vi "sub_ofdm_mes_ce.vi"(11 "ZF channel estimates":cdb[](array[numeric])) -> (3 "interpolated mes carrier CE":cdb[](array[numeric]))   [LabVIEW 2014]
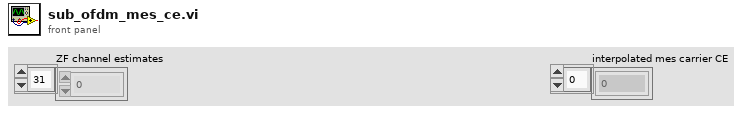
[diagram p1: front panel]
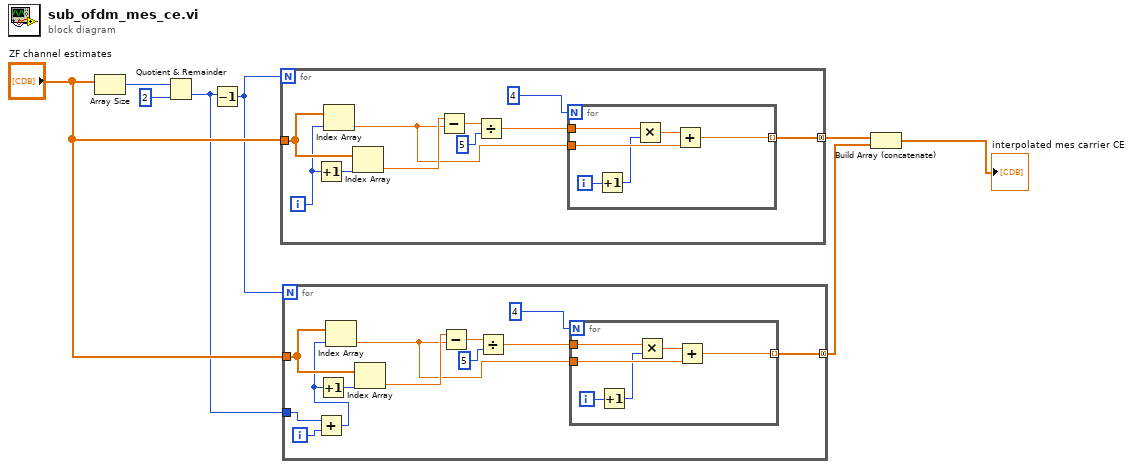
[diagram p0: block diagram]
diagram:
  n1 = Array Size(array="ZF channel estimates") -> (size(s)=w8:i32)
  n2 = Quotient & Remainder(x=w8, y=2) -> (floor(x/y)=w4:i32)  [unwired: 1 out]
  n3 = Decrement(x=w4) -> (x-1=w5:i32)
  n4 = for {
    N: w5 -> [_]
    tunnel: "ZF channel estimates" -> [w18]
    tunnel: [w9] -> w3 mode=concatenating
    i -> [w17]
    n5 = Increment(x=w17) -> (x+1=w16:i32)
    n6 = Index Array(array=w18, index=w17) -> (element=w10:cdb)
    n7 = Index Array(array=w18, index=w16) -> (element=w15:cdb)
    n8 = Subtract(x=w15, y=w10) -> (x-y=w14:cdb)
    n9 = Divide(x=w14, y=5) -> (x/y=w11:cdb)
    n10 = for {
      N: 4 -> [_]
      tunnel: w11 -> [w24]
      tunnel: w10 -> [w22]
      tunnel: [w19] -> w9 mode=indexing
      i -> [w21]
      n11 = Increment(x=w21) -> (x+1=w20:i32)
      n12 = Multiply(x=w24, y=w20) -> (x*y=w23:cdb)
      n13 = Add(x=w23, y=w22) -> (x+y=w19:cdb)
    }
  }
  n14 = for {
    N: w5 -> [_]
    tunnel: "ZF channel estimates" -> [w36]
    tunnel: [w28] -> w2 mode=concatenating
    tunnel: w4 -> [w26]
    i -> [w27]
    n15 = Add(x=w26, y=w27) -> (x+y=w25:i32)
    n16 = Increment(x=w25) -> (x+1=w35:i32)
    n17 = Index Array(array=w36, index=w25) -> (element=w29:cdb)
    n18 = Index Array(array=w36, index=w35) -> (element=w34:cdb)
    n19 = Subtract(x=w34, y=w29) -> (x-y=w33:cdb)
    n20 = Divide(x=w33, y=5) -> (x/y=w30:cdb)
    n21 = for {
      N: 4 -> [_]
      tunnel: w30 -> [w42]
      tunnel: w29 -> [w40]
      tunnel: [w37] -> w28 mode=indexing
      i -> [w39]
      n22 = Increment(x=w39) -> (x+1=w38:i32)
      n23 = Multiply(x=w42, y=w38) -> (x*y=w41:cdb)
      n24 = Add(x=w41, y=w40) -> (x+y=w37:cdb)
    }
  }
  n25 = Build Array (concatenate)(w3, w2) -> (→"interpolated mes carrier CE":cdb[])
